vi "Exemple_Metrics_Roc_Auc_Score.vi"() -> ()   [LabVIEW 2020]
uses:
  Objet/3 - Model selection and evaluation/3.3 - Metrics and scoring/roc_auc_score/Roc_Auc_Score.vi
panel:
  out "Score":string
  out "error out":errorcluster caption="sortie d'erreur"
  in  "roc_auc_score":T1={"average"="macro", "sample_weight"=[], "max_fpr"="None", "multi_class"="raise", "labels"=["None"]}
  in  "error in (no error)":errorcluster caption="entrée d'erreur (pas d'erreur)"
  in  "y_score":string[][](array[string])=[["0,1"], ["0,4"], ["0,35"], ["0,8"]]
  in  "y_true":string[][](array[string])=[["0"], ["0"], ["1"], ["1"]]
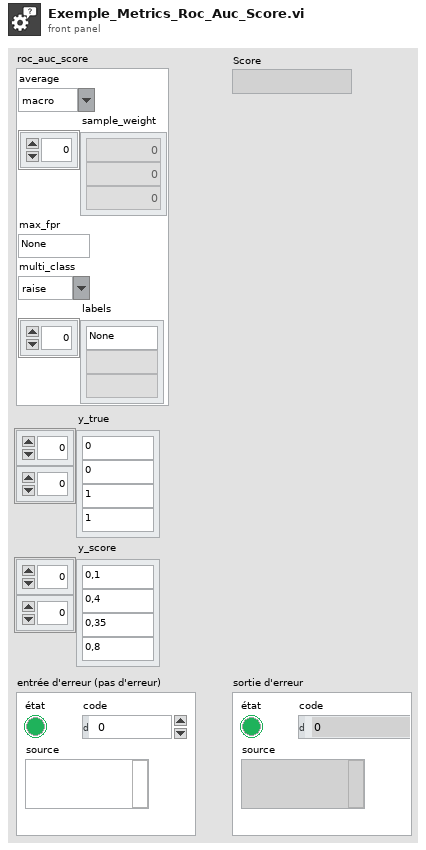
[diagram p1: front panel]
types:
  T1 = cluster{"average":string, "sample_weight":dbl[], "max_fpr":string, "multi_class":string, "labels":string[]}
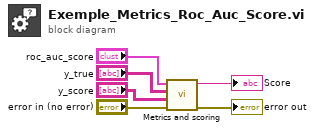
[diagram p0: block diagram]
diagram:
  n1 = call-poly "Metrics and scoring.vi"("error in (no error)"="error in (no error)", "y_score"="y_score", "y_true"="y_true", "roc_auc_score"="roc_auc_score") -> ("error out"=→"error out":errorcluster, "Score"=→"Score":string)  [unwired: 6 in]
